vi "Set Dependent Modules.vi"(8 "error in (no error)":errorcluster, 10 "Dependent Module Refs":T1[](array[typedef]) format="%.0x", 11 "Routing and Faulting Ref in":T1 format="%.0x") -> (0 "error out":errorcluster, 3 "Routing and Faulting Ref out":T1 format="%.0x")   [LabVIEW 2017, in "Routing and Faulting System Explorer.lvlib"]
uses:
  Routing and Faulting System Explorer.lvlib
  <vilib>/NI Veristand/Custom Device API/Custom Device Item Ref.ctl
  <vilib>/NI Veristand/Custom Device API/Get Item Property (String Array).vi
  <vilib>/NI Veristand/Custom Device API/Set Item Property (Dependent Node Pointer).vi
  <vilib>/NI Veristand/Custom Device API/Set Item Property (String Array).vi
  <vilib>/NI Veristand/Custom Device API/Custom Device API.lvlib
  Shared/Routing and Faulting Hardware API/Routing and Faulting Hardware API.lvlib
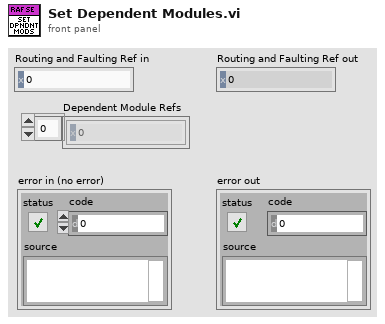
[diagram p1: front panel]
types:
  T1 = typedef "Custom Device API.lvlib/Custom Device Item Ref.ctl" = u64
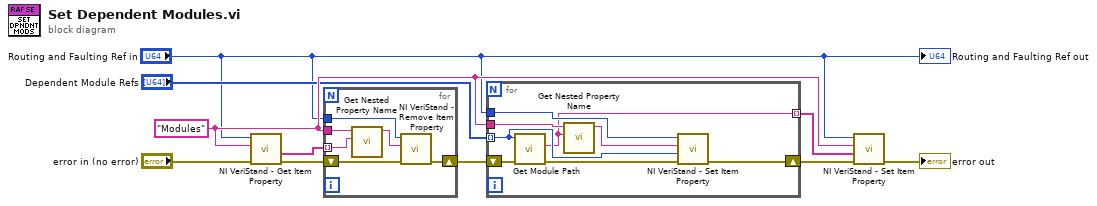
[diagram p0: block diagram]
diagram:
  w10 = "Modules" ("string")
  n1 = call-poly <vilib>:"NI VeriStand - Get Item Property.vi"("error in (no error)"="error in (no error)", "Property Name"=w10, "Item Ref in"="Routing and Faulting Ref in") -> ("error out"=w8:errorcluster, "Value"=w9:string[])  [unwired: 5 in, 2 out]
  n2 = for {
    shift-right: [w14] -> w2
    shift-left: w8 -> [w15]
    tunnel: "Routing and Faulting Ref in" -> [w13]
    tunnel: w10 -> [w12]
    tunnel: w9 -> [w11] mode=indexing
    n3 = call "Get Nested Property Name.vi"("property key name"=w11, "property base name"=w12) -> ("full property name"=w16:string)  [unwired: 9 in]
    n4 = call <vilib>:"NI VeriStand - Remove Item Property.vi"("error in (no error)"=w15, "Property Name"=w16, "Item Ref in"=w13) -> ("error out"=w14:errorcluster)  [unwired: 6 in, 2 out]
  }
  n5 = for {
    shift-right: [w21] -> w4
    shift-left: w2 -> [w19]
    tunnel: "Routing and Faulting Ref in" -> [w22]
    tunnel: w10 -> [w23]
    tunnel: "Dependent Module Refs" -> [w20] mode=indexing
    tunnel: [w17] -> w6 mode=indexing
    n6 = call "Get Module Path.vi"("error in (no error)"=w19, "Hardware Ref in"=w20) -> ("error out"=w18:errorcluster, "Resource"=w17:string)  [unwired: 6 in, 2 out]
    n7 = call "Get Nested Property Name.vi"("property key name"=w17, "property base name"=w23) -> ("full property name"=w24:string)  [unwired: 9 in]
    n8 = call-poly <vilib>:"NI VeriStand - Set Item Property.vi"("error in (no error)"=w18, "Dependent Node Ref"=w20, "Property Name"=w24, "Item Ref in"=w22) -> ("error out"=w21:errorcluster)  [unwired: 5 in, 2 out]
  }
  n9 = call-poly <vilib>:"NI VeriStand - Set Item Property.vi"("error in (no error)"=w4, "Value"=w6, "Property Name"=w10, "Item Ref in"="Routing and Faulting Ref in") -> ("error out"=→"error out":errorcluster)  [unwired: 5 in, 2 out]
  "Routing and Faulting Ref out" <- "Routing and Faulting Ref in"
